vi "CRYFlatten Limits.vi"(11 "Limits":T1={"Name"="", "Tolerance"=2, "X Axis"=1, "Limits"=2, "Upper Limit"=[{100.0, 1.0}, {1000.0, 1.0}], "Align Ref"={1000.0, 0.0}, "Lower Limit"=[{100.0, -1.0}, {1000.0, -1.0}], "Y data"=1, "Y unit"="(und)", "Y dB ref"=1.0, "Curve Names"=[], "Y-Resolution"=1, "Type"=1, "x float"=FALSE, "X min-max-step"={"Limit X Offset Min"=0.9, "Limit X Offset Max"=1.1, "Limit X Offset Step Size"=1.01}, "magn/phase"=1, "Upper Limit Type"=0, "Lower Limit Type"=0, "Lim Curve axis up"=1, "Lim Curve axis lo"=1, "Data Selection Upper"=1, "Data Selection Lower"=1, "X-Resolution"=1, "Output failed point curves?"=FALSE, "X data"=1, "X unit"="(und)", "X dB ref"=1.0, "X-Y Graph Set-up"="", "Tab Value"=enum."Parameters", "Help"="", "X Up Val"=0.0, "Y Up Val"=0.0, "X Low Val"=0.0, "Y Low Val"=0.0, "Up Limit Val"=0.0, "Low Limit Val"=0.0, "bAdd DataName"=FALSE, "Custom Name"=""} {"X data" items=["dB", "Lin"]; "Data Selection Lower" items=["Single Values", "Curves", "Waveforms"]; "Data Selection Upper" items=["Single Values", "Curves", "Waveforms"]; "Lim Curve axis lo" items=["x", "y", "z"]; "Lim Curve axis up" items=["x", "y", "z"]; "Lower Limit Type" items=["User Defined", "Memory List"]; "Upper Limit Type" items=["User Defined", "Memory List"]; "Type" items=["Single Value", "Curve", "Waveforms", "Voltmeter"]; "Y data" items=["dB", "Lin"]; "Limits" items=["Upper Only", "Lower Only", "Upper & Lower"]; "X Axis" items=["Linear", "Logarithmic"]; "Tolerance" items=["Individual Points", "Absolute Limits", "Floating Limits", "Floating Data", "Aligned Limits", "Aligned Data"]}) -> (3 "Flatten Limits String":string)   [LabVIEW 2013]
uses:
  Typedef Control/CRYLimits.ctl
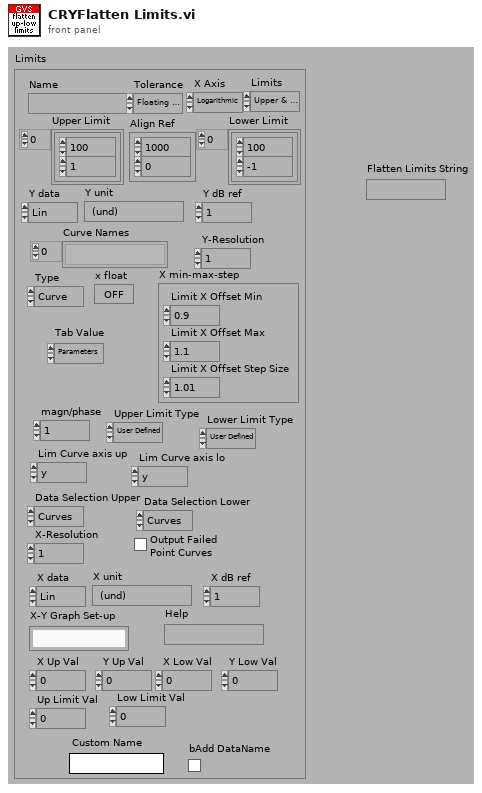
[diagram p1: front panel]
types:
  T1 = typedef "CRYLimits.ctl" = cluster{"Name":string, "Tolerance":u16, "X Axis":u16, "Limits":u16, "Upper Limit":cluster{dbl, dbl}[], "Align Ref":cluster{dbl, dbl}, "Lower Limit":cluster{dbl, dbl}[], "Y data":u16, "Y unit":string, "Y dB ref":dbl, "Curve Names":string[], "Y-Resolution":u8, "Type":u16, "x float":bool, "X min-max-step":cluster{"Limit X Offset Min":dbl, "Limit X Offset Max":dbl, "Limit X Offset Step Size":dbl}, "magn/phase":u16, "Upper Limit Type":u16, "Lower Limit Type":u16, "Lim Curve axis up":u16, "Lim Curve axis lo":u16, "Data Selection Upper":u16, "Data Selection Lower":u16, "X-Resolution":u8, "Output failed point curves?":bool, "X data":u16, "X unit":string, "X dB ref":dbl, "X-Y Graph Set-up":string, "Tab Value":enum32{"Data", "Parameters"}, "Help":string, "X Up Val":dbl, "Y Up Val":dbl, "X Low Val":dbl, "Y Low Val":dbl, "Up Limit Val":dbl, "Low Limit Val":dbl, "bAdd DataName":bool, "Custom Name":string}
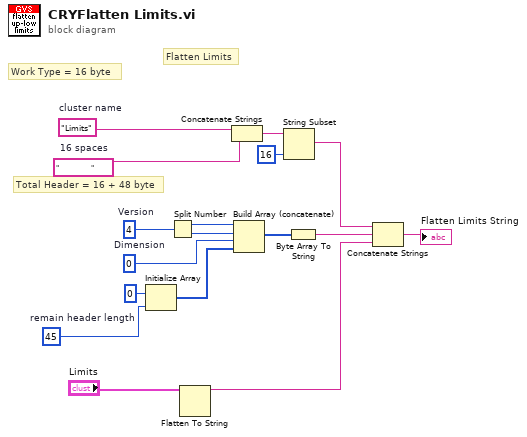
[diagram p0: block diagram]
diagram:
  w2 = "                "  # 16 spaces
  w3 = "Limits"  # cluster name
  w8 = u16 4  # Version
  w11 = u8 0  # Dimension
  w7 = 45  # remain header length
  # "Flatten Limits"
  # "Work Type = 16 byte"
  # "Total Header = 16 + 48 byte"
  n1 = Initialize Array(u8 0 ("element"), w7) -> (w13:u8[])
  n2 = Split Number(x=w8) -> (hi(x)=w9:u8, lo(x)=w10:u8)
  n3 = Flatten To String(anything="Limits") -> (data string=w14:string)  [unwired: 1 in, 4 out]
  n4 = Concatenate Strings(w3, w2) -> (w4:string)
  n5 = Build Array (concatenate)(w9, w10, w11, w13) -> (w12:u8[])
  n6 = String Subset(string=w4, length (rest)=16 ("length (rest)")) -> (substring=w16:string)  [unwired: 1 out]
  n7 = Byte Array To String(unsigned byte array=w12) -> (string=w15:string)
  n8 = Concatenate Strings(w16, w15, w14) -> (→"Flatten Limits String":string)
